vi "date_formatting_test.vi"() -> ()   [LabVIEW 2010]
panel:
  out "String":string
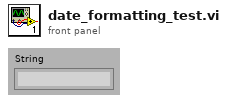
[diagram p1: front panel]
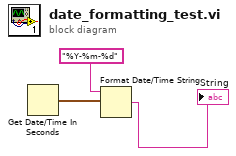
[diagram p0: block diagram]
diagram:
  n1 = Get Date/Time In Seconds() -> (seconds since 1Jan1904=w3:timestamp)
  n2 = Format Date/Time String(time format string (%c)="%Y-%m-%d", seconds (now)=w3) -> (date/time string=→"String":string)  [unwired: 1 in]
